vi "Add JobName.vi"(9 "Job Target":string, 10 "Data in":variant, 11 "Build Job in":refnum<class "Build Job.lvclass">) -> (1 "Job Name":string, 2 "Data Out":variant)   [LabVIEW 2014, in "Build Job.lvclass"]
uses:
  Build Job.lvclass
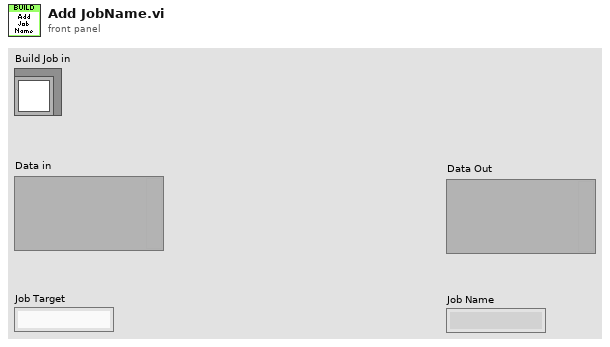
[diagram p1: front panel]
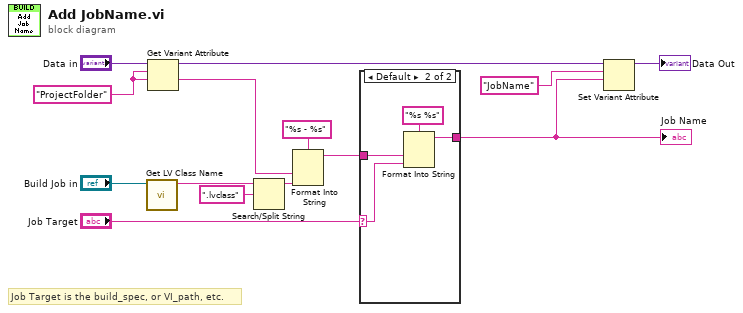
[diagram p0: block diagram]
diagram:
  w7 = "ProjectFolder" ("input 1")
  # "Job Target is the build_spec, or VI_path, etc."
  n1 = call <vilib>:"Get LV Class Name.vi"("object"="Build Job in") -> ("class name"=w3:string)  [unwired: 9 in, 1 out]
  n2 = Get Variant Attribute(Variant="Data in", name=w7, default value (empty Variant)=w7) -> (duplicate Variant=w6:variant, value=w8:string)  [unwired: 1 in, 2 out]
  n3 = Search/Split String(string=w3, search string/char (-)=".lvclass") -> (substring before match=w2:string)  [unwired: 1 in, 2 out]
  n4 = Format Into String(format string="%s - %s", w8, w2) -> (resulting string=w12:string)  [unwired: 2 in, 1 out]
  n5 = case shown="Default" "Job Target" {
    selector: "Job Target" -> [_ w16]
    tunnel: w12 -> [w15 w18]
    tunnel: [w15 w17] -> w11
    frame "" {
    }
    frame Default {
      n6 = Format Into String(format string="%s %s", w18, w16) -> (resulting string=w17:string)  [unwired: 2 in, 1 out]
    }
  }
  "Job Name" <- w11
  n7 = Set Variant Attribute(Variant=w6, name="JobName", value=w11) -> (Variant out=→"Data Out":variant)  [unwired: 1 in, 2 out]
